vi "CalInjectRT.vi"(7 "Boolean in":refnum<vi>, 8 "error in (no error)":errorcluster, 11 "MotorStateIn":enum16{"Open", "Moving", "Close", "Wait"}(ring)) -> (0 "error out":errorcluster, 3 "MotorStateOut":enum16{"Open", "Moving", "Close", "Wait"}(ring))   [LabVIEW 2016]
uses:
  controls/ColorStates.ctl
  controls/RT-Variables.lvlib
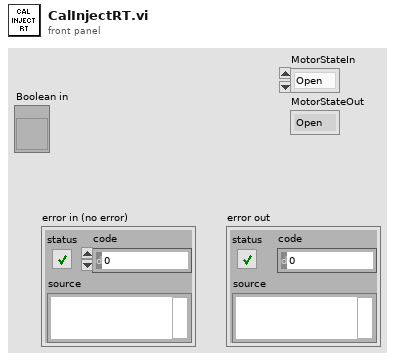
[diagram p1: front panel]
types:
  T1 = typedef "RT-Variables.lvlib/ColorStates.ctl" = enum16{"Red", "Yellow", "Green"}
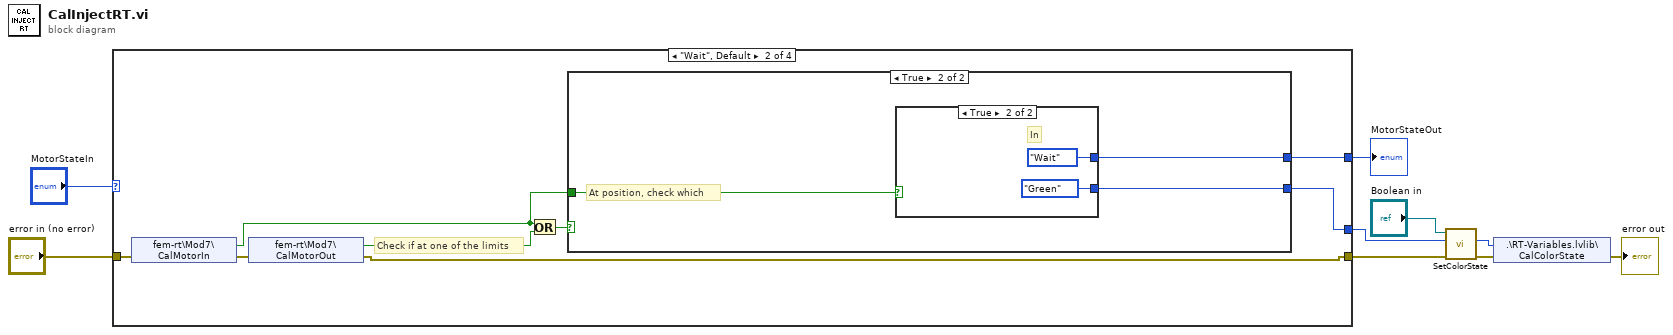
[diagram p0: block diagram]
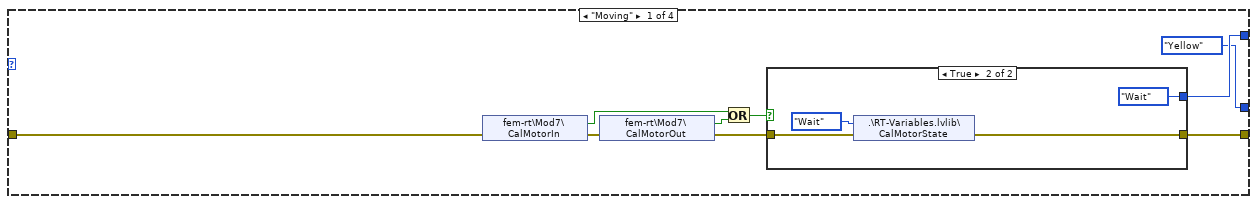
[diagram p2: hidden frame]
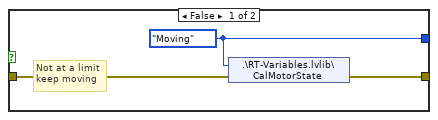
[diagram p3: hidden frame]
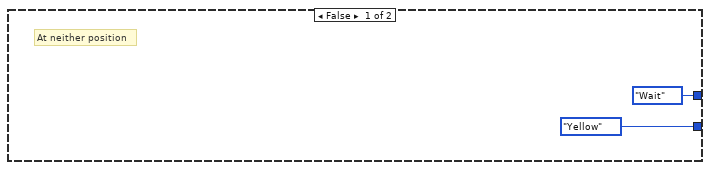
[diagram p4: hidden frame]
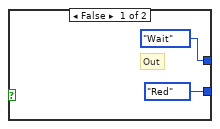
[diagram p5: hidden frame]
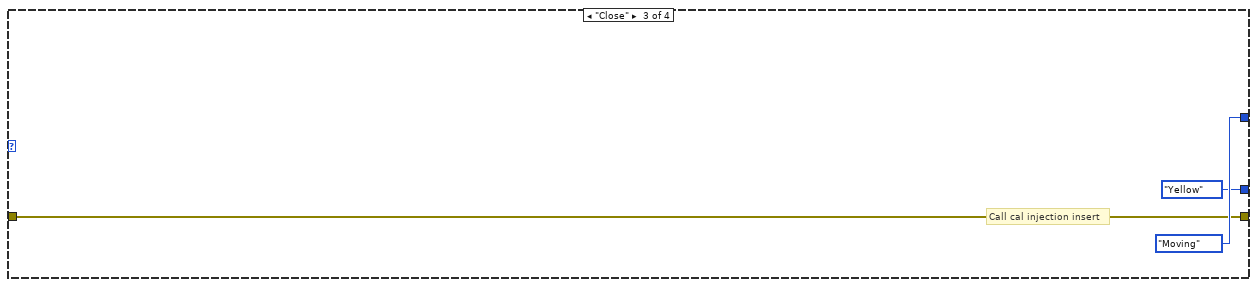
[diagram p6: hidden frame]
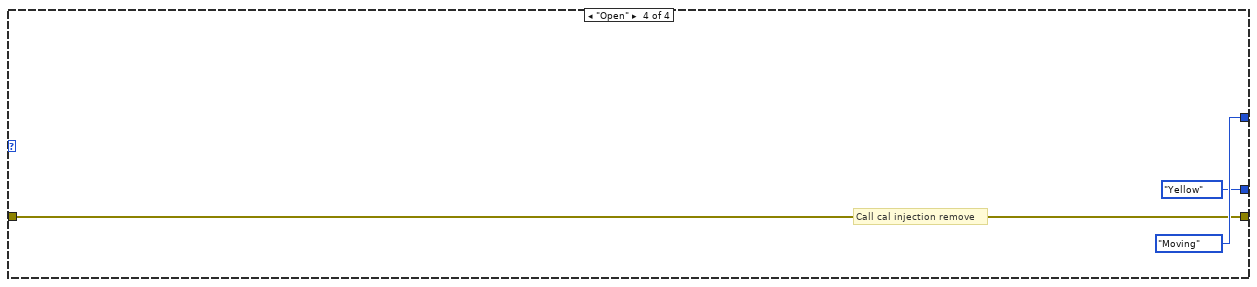
[diagram p7: hidden frame]
diagram:
  n1 = case shown="\"Wait\", Default" "MotorStateIn" {
    tunnel: [w14 w29 w43 w46] -> w4
    tunnel: "error in (no error)" -> [w11 w33 w43 w46]
    tunnel: [w12 w32 enum16{"Open", "Moving", "Close", "Wait"}."Moving" ("CoverState") enum16{"Open", "Moving", "Close", "Wait"}."Moving" ("CoverState")] -> w7
    tunnel: [ColorStates."Yellow" ("ColorStateOut") w31 ColorStates."Yellow" ("ColorStateOut") ColorStates."Yellow" ("ColorStateOut")] -> w5
    frame "Moving" {
      n2 = shared-variable "fem-rt\\Mod7\\CalMotorIn"(error in=w11) -> (w17:bool, error out=w13:errorcluster)
      n3 = shared-variable "fem-rt\\Mod7\\CalMotorOut"(error in=w13) -> (w16:bool, error out=w15:errorcluster)
      n4 = Or(x=w17, y=w16) -> (x .or. y?=w18:bool)
      n5 = case shown="True" w18 {
        tunnel: w15 -> [w21 w25]
        tunnel: [w20 w22] -> w14
        tunnel: [w19 enum16{"Open", "Moving", "Close", "Wait"}."Wait" ("CoverState")] -> w12
        frame False {
          w19 = enum16{"Open", "Moving", "Close", "Wait"}."Moving" ("CoverState")
          # "Not at a limit\nkeep moving"
          n6 = shared-variable ".\\RT-Variables.lvlib\\CalMotorState"(w19, error in=w21) -> (error out=w20:errorcluster)
        }
        frame True {
          n7 = shared-variable ".\\RT-Variables.lvlib\\CalMotorState"(enum16{"Open", "Moving", "Close", "Wait"}."Wait" ("CoverState"), error in=w25) -> (error out=w22:errorcluster)
        }
      }
    }
    frame "Wait", Default {
      # "Check if at one of the limits"
      n8 = shared-variable "fem-rt\\Mod7\\CalMotorIn"(error in=w33) -> (w26:bool, error out=w30:errorcluster)
      n9 = shared-variable "fem-rt\\Mod7\\CalMotorOut"(error in=w30) -> (w28:bool, error out=w29:errorcluster)
      n10 = Or(x=w26, y=w28) -> (x .or. y?=w27:bool)
      n11 = case shown="True" w27 {
        tunnel: [enum16{"Open", "Moving", "Close", "Wait"}."Wait" ("CoverState") w38] -> w32
        tunnel: [ColorStates."Yellow" ("ColorStateOut") w37] -> w31
        tunnel: w26 -> [_ w36]
        frame False {
          # "At neither position"
        }
        frame True {
          # "At position, check which"
          n12 = case shown="True" w36 {
            tunnel: [enum16{"Open", "Moving", "Close", "Wait"}."Wait" ("CoverState") enum16{"Open", "Moving", "Close", "Wait"}."Wait" ("CoverState")] -> w38
            tunnel: [ColorStates."Red" ("ColorStateOut") ColorStates."Green" ("ColorStateOut")] -> w37
            frame False {
              # "Out"
            }
            frame True {
              # "In"
            }
          }
        }
      }
    }
    frame "Close" {
      # "Call cal injection insert"
    }
    frame "Open" {
      # "Call cal injection remove"
    }
  }
  "MotorStateOut" <- w7
  n13 = call "SetColorState.vi"("error in (no error)"=w4, "ColorStateIn"=w5, "Boolean in"="Boolean in") -> ("error out"=w2:errorcluster, "ColorStateOut"=w3:T1)  [unwired: 7 in]
  n14 = shared-variable ".\\RT-Variables.lvlib\\CalColorState"(w3, error in=w2) -> (error out=→"error out":errorcluster)
